vi "output_enable.vi"(8 "error in (no error)":errorcluster, 9 "Enable":bool, 10 "Channel":string="1", 11 "VISA Refnum in":refnum<visa-resource-name>) -> (0 "error out":errorcluster, 3 "VISA Refnum out":refnum<visa-resource-name>)   [LabVIEW 2018, in "Aim-TTi PL303-P.lvlib"]
uses:
  <instrlib>/Aim-TTi PL303-P/Aim-TTi PL303-P.lvlib
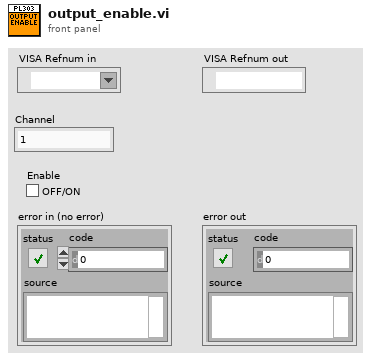
[diagram p1: front panel]
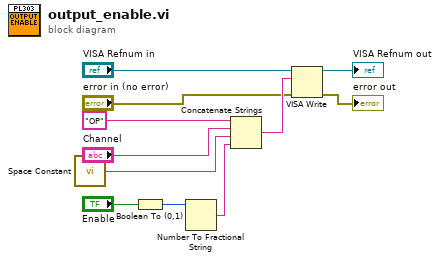
[diagram p0: block diagram]
diagram:
  n1 = call <vilib>:"Space Constant.vi"() -> ("String"=w4:string)
  n2 = Boolean To (0,1)(Boolean="Enable") -> (0, 1=w2:i16)
  n3 = Number To Fractional String(number=w2) -> (F-format string=w3:string)  [unwired: 3 in]
  n4 = Concatenate Strings("OP" ("string"), "Channel", w4, w3) -> (w9:string)
  n5 = VISA Write(VISA resource name="VISA Refnum in", write buffer=w9, error in (no error)="error in (no error)") -> (VISA resource name out=→"VISA Refnum out":refnum<visa-resource-name>, error out=→"error out":errorcluster)  [unwired: 1 out]
